vi "Get Plugin Directorys.vi"(8 "error in":errorcluster) -> (0 "error out":errorcluster, 2 "Creation Success":bool[](array[boolean]), 3 "Plugin Directories":path[](array[path]))   [LabVIEW 2020, in "RxnRover.lvlib" / "Plugin Manager.lvlib"]
doc: "Returns an array of plugin directories, creating each plugin directory that does not already exist. The plugin directories are determined by the Get Default Plugin Directories VI. An array of booleans parallel to the plugin directories array is also returned, indicating whether each directory was successfully created or already exists (True) or failed to be created (False)."
uses:
  Plugin Manager.lvlib
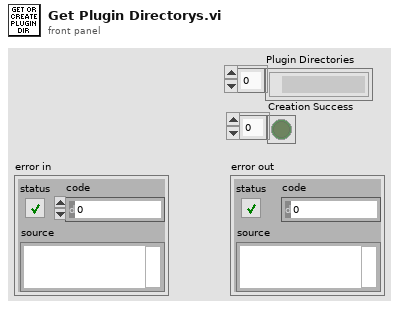
[diagram p1: front panel]
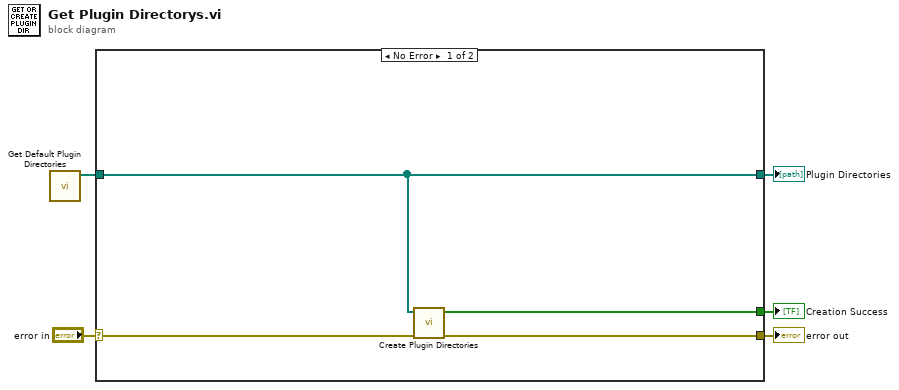
[diagram p0: block diagram]
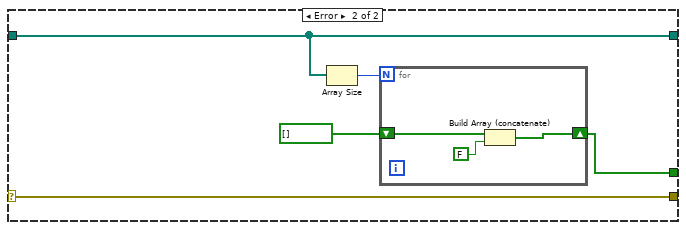
[diagram p2: hidden frame]
diagram:
  n1 = call "Get Default Plugin Directories.vi"() -> ("Default Plugin Directories"=w2:path[])  [unwired: 11 in]
  n2 = case shown="No Error" "error in" {
    selector: "error in" -> [w8 w14]
    tunnel: [w9 w14] -> w5
    tunnel: [w6 w10] -> w1
    tunnel: w2 -> [w7 w12]
    tunnel: [w7 w12] -> w3
    frame No Error {
      n3 = call "Create Plugin Directories.vi"("error in (no error)"=w8, "Plugin Directory Array"=w7) -> ("error out"=w9:errorcluster, "Creation Success"=w6:bool[])  [unwired: 8 in]
    }
    frame Error {
      n4 = Array Size(array=w12) -> (size(s)=w13:i32)
      n5 = for {
        N: w13 -> [_]
        shift-right: [w16] -> w10
        shift-left: bool[] [] ("Creation Success") -> [w17]
        n6 = Build Array (concatenate)(w17, FALSE) -> (w16:bool[])
      }
    }
  }
  "error out" <- w5
  "Plugin Directories" <- w3
  "Creation Success" <- w1
